vi "CSTK_BuildApplication_Manager_Package_Zip.vi"(5 "Files Generated by Build":path[](array[path]) caption="通过生成创建的文件", 7 "Destination Path":path caption="目标路径", 8 "error in (no error)":errorcluster caption="错误输入（无错误）", 10 "Build Specification Name":string caption="程序生成规范名称") -> (0 "error out":errorcluster caption="错误输出")   [LabVIEW 2015, in "CSTK_BuildApplication_Manager.lvlib"]
uses:
  CSTK_BuildApplication_Manager.lvlib
  CSTK_BuildApplication_Manager_data.ctl
  CSTK_BuildApplication_Manager_selector.ctl
  user32.dll
panel:
  in  "根据版本号修改EXE文件名":bool
  in  "打包成ZIP文件？":bool=TRUE
  in  "确定按钮":bool
  in  "注释":string
  # "Build Application Manager"
  # "输入版本修改日志"
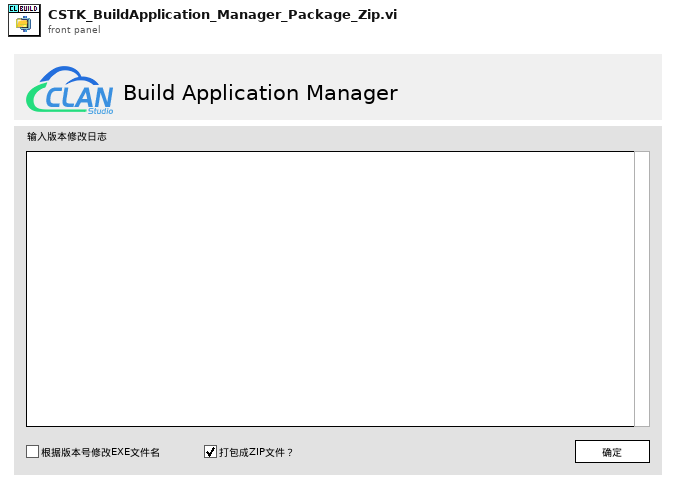
[diagram p1: front panel]
types:
  T1 = typedef "CSTK_BuildApplication_Manager.lvlib/CSTK_BuildApplication_Manager_data.ctl" = cluster{"Build Specification Name":string, "Destination Path":path, "Files Generated by Build":path[], "Exe Path Generated by Build":path, "Version":string, "Datatime":timestamp, "ChangeLog":string, "Package as a ZIP file?":bool, "Rename EXE File Name?":bool, "Zip File Path":path}
  T2 = enum32{"Invalid", "Standard", "Closed", "Hidden", "Minimized", "Maximized"}
  T3 = typedef "CSTK_BuildApplication_Manager.lvlib/CSTK_BuildApplication_Manager_selector.ctl" = cluster{"Package as a ZIP file?":bool, "Rename EXE File Name?":bool}
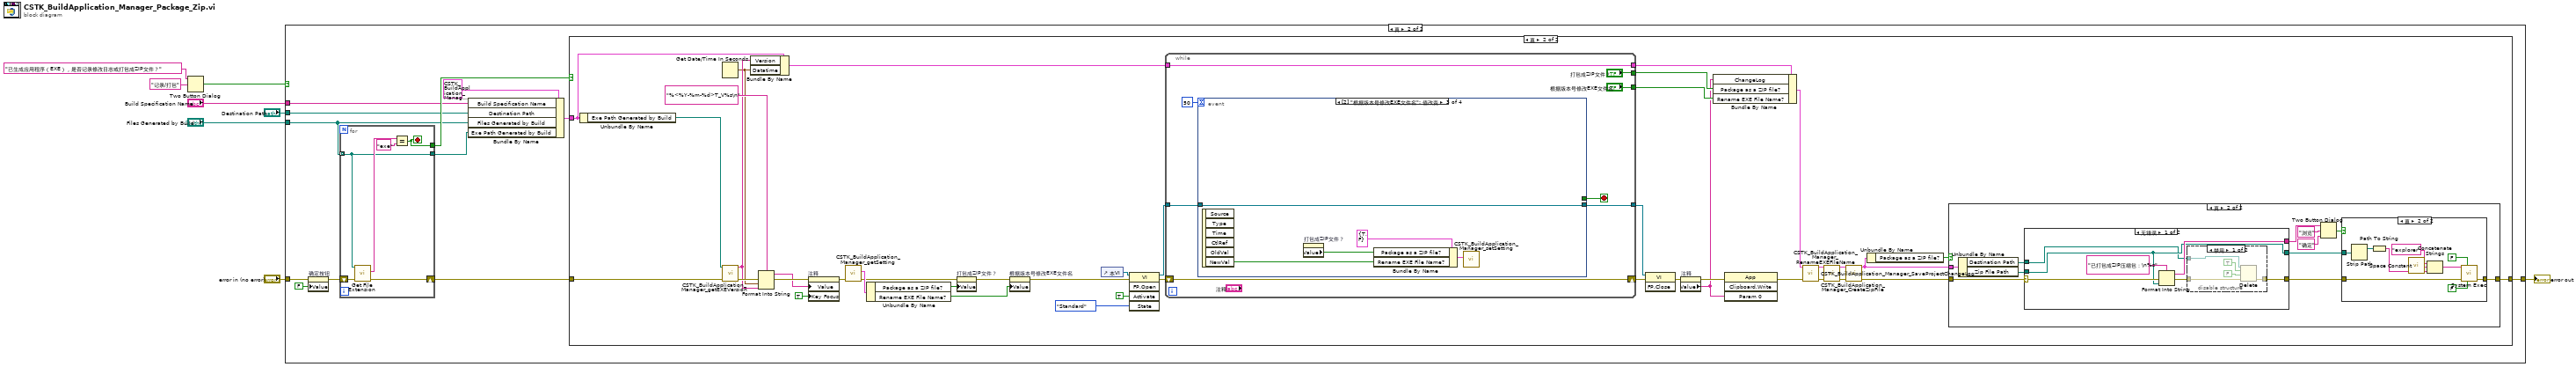
[diagram p0: block diagram]
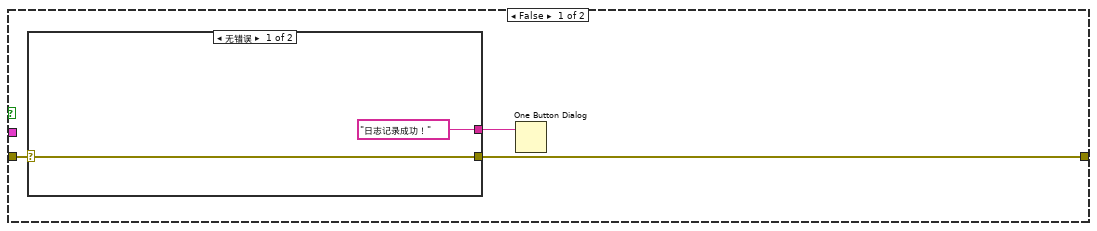
[diagram p4: hidden frame]
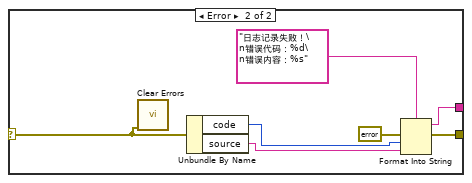
[diagram p5: hidden frame]
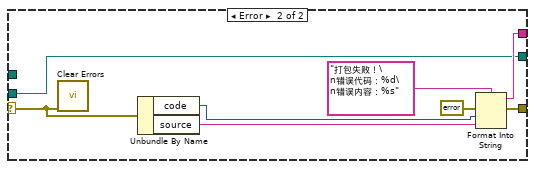
[diagram p8: hidden frame]
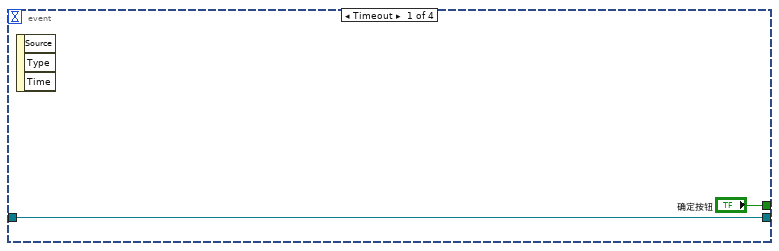
[diagram p9: hidden frame]
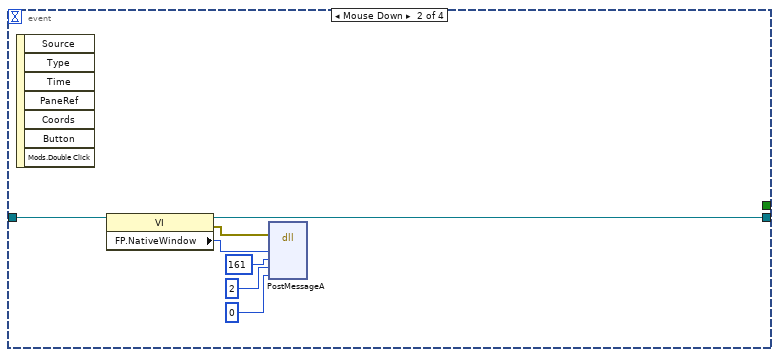
[diagram p10: hidden frame]
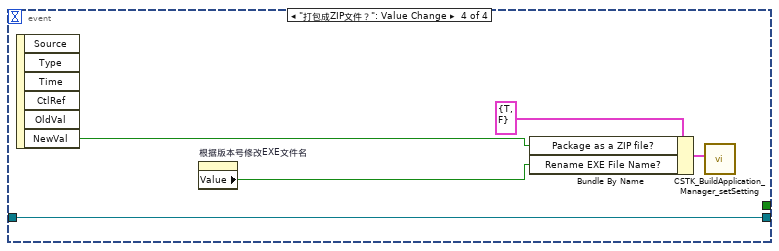
[diagram p11: hidden frame]
diagram:
  n1 = Two Button Dialog(message="已生成应用程序（EXE），是否记录修改日志或打包成ZIP文件？" ("消息"), 2:"记录/打包" ("T按钮名称（“确定”）")) -> (T button?=w1:bool)  [unwired: 1 in]
  n2 = case shown="真" w1 {
    tunnel: "Files Generated by Build" -> [_ w12]
    tunnel: "error in (no error)" -> [w9 w20]
    tunnel: [w9 w21] -> w5
    tunnel: "Build Specification Name" -> [_ w14]
    tunnel: "Destination Path" -> [_ w13]
    frame False {
    }
    frame True {
      n3 = property on="确定按钮" class="Bool (严格)"(error in=w20, "Value"=FALSE ("确定按钮")) -> (error out=w18:errorcluster)  [unwired: 1 in, 1 out]
      n4 = for {
        tunnel: w12 -> [w148] mode=indexing
        shift-right: [w146] -> w17
        shift-left: w18 -> [w151]
        tunnel: [w148] -> w11
        tunnel: [w147] -> w16
        stop <- w147 stop-if-true
        n5 = call <vilib>:"Get File Extension.vi"("error in (no error)"=w151, "file"=w148) -> ("error out"=w146:errorcluster, "lowercase file extension"=w150:string)  [unwired: 5 in, 3 out]
        n6 = Equal?(x=w150, y="exe") -> (x = y?=w147:bool)
      }
      n7 = Bundle By Name(cluster=T1 {"Build Specification Name"="", "Destination Path"=path "", "Files Generated by Build"=[], "Exe Path Generated by Build"=path "", "Version"="", "Datatime"=timestamp(0 s since 1904-01-01), "ChangeLog"="", "Package as a ZIP file?"=TRUE, "Rename EXE File Name?"=FALSE, "Zip File Path"=path ""} ("BuildApplication Data"), "Build Specification Name"=w14, "Destination Path"=w13, "Files Generated by Build"=w12, "Exe Path Generated by Build"=w11) -> (w10:T1)
      n8 = case shown="真" w16 {
        tunnel: [w22 w63] -> w21
        tunnel: w17 -> [w22 w62]
        tunnel: w10 -> [_ w44]
        frame False {
        }
        frame True {
          n9 = Unbundle By Name(w44) -> ("Exe Path Generated by Build"=w45:path)
          n10 = Get Date/Time In Seconds() -> (seconds since 1Jan1904=w42:timestamp)
          n11 = call "CSTK_BuildApplication_Manager_getEXEVersion.vi"("错误输入（无错误）"=w62, "EXE路径"=w45) -> ("错误输出"=w55:errorcluster, "版本号"=w43:string)  [unwired: 8 in]
          n12 = Bundle By Name(cluster=w44, "Version"=w43, "Datatime"=w42) -> (w41:T1)
          n13 = Format Into String(format string="%<%Y-%m-%d>T_V%s\n" ("格式字符串"), error in=w55, w42, w43) -> (resulting string=w53:string, error out=w54:errorcluster)  [unwired: 1 in]
          n14 = property on="注释" class="Str"(error in=w54, "Value"=w53, "Key Focus"=TRUE ("键选中")) -> (error out=w29:errorcluster)  [unwired: 1 in, 1 out]
          n15 = call "CSTK_BuildApplication_Manager_getSetting.vi"("Error in"=w29) -> ("Error out"=w23:errorcluster, "BuildApplication Selector"=w28:T3)  [unwired: 8 in, 1 out]
          n16 = Unbundle By Name(w28) -> ("Package as a ZIP file?"=w27:bool, "Rename EXE File Name?"=w26:bool)
          n17 = property on="打包成ZIP文件？" class="Bool (严格)"(error in=w23, "Value"=w27) -> (error out=w25:errorcluster)  [unwired: 1 in, 1 out]
          n18 = property on="根据版本号修改EXE文件名" class="Bool (严格)"(error in=w25, "Value"=w26) -> (error out=w24:errorcluster)  [unwired: 1 in, 1 out]
          n19 = control-ref of="本VI"() -> (w57:refnum<vi>)
          n20 = invoke class="VI" method="FP.Open"(reference=w57, error in=w24, "Activate"=TRUE ("激活？"), "State"=T2."Standard" ("状态")) -> (reference out=w47:refnum<vi>, error out=w59:errorcluster)  [unwired: 1 in, 3 out]
          n21 = while {
            shift-right: [w126] -> w58
            shift-left: w59 -> [w126]
            tunnel: ["打包成ZIP文件？"] -> w39
            tunnel: ["根据版本号修改EXE文件名"] -> w38
            tunnel: w47 -> [w120]
            tunnel: [w121] -> w46
            tunnel: w41 -> [w119]
            tunnel: [w119] -> w40
            stop <- w122 stop-if-true
            n22 = event shown="[2] \"根据版本号修改EXE文件名\": 值改变" {
              selector: _ -> [_ _ _ _]
              dyn-events: _ -> [_ _ _ _]
              timeout: 50 -> [_ _ _ _]
              tunnel: ["确定按钮" _ _ _] -> w122
              tunnel: [w127 w129 w140 w145] -> w121
              tunnel: w120 -> [w127 w130 w140 w145]
              event Timeout {
                n23 = event-data() -> ()  [unwired: 1 in, 3 out]
              }
              event Mouse Down {
                n24 = event-data() -> ()  [unwired: 1 in, 7 out]
                n25 = property class="VI"(reference=w130) -> (reference out=w129:refnum<vi>, error out=w131:errorcluster, "FP.NativeWindow"=w132:u64)  [unwired: 1 in]
                n26 = dll-call lib="user32.dll" fn="PostMessageA"(error in=w131, "hWnd"=w132, "Msg"=161, "wParam"=2, "IParam"=0 ("wParam")) -> ()  [unwired: 7 in, 2 out]
              }
              event "根据版本号修改EXE文件名": Value Change {
                n27 = event-data() -> ("NewVal"=w137:bool)  [unwired: 1 in, 5 out]
                n28 = property on="打包成ZIP文件？" class="Bool (严格)"() -> ("Value"=w136:bool)  [unwired: 2 in, 2 out]
                n29 = Bundle By Name(cluster=T3 {"Package as a ZIP file?"=TRUE, "Rename EXE File Name?"=FALSE} ("BuildApplication Selector"), "Package as a ZIP file?"=w136, "Rename EXE File Name?"=w137) -> (w138:T3)
                n30 = call "CSTK_BuildApplication_Manager_setSetting.vi"("BuildApplication Selector"=w138) -> ()  [unwired: 10 in, 1 out]
              }
              event "打包成ZIP文件？": Value Change {
                n31 = event-data() -> ("NewVal"=w141:bool)  [unwired: 1 in, 5 out]
                n32 = property on="根据版本号修改EXE文件名" class="Bool (严格)"() -> ("Value"=w142:bool)  [unwired: 2 in, 2 out]
                n33 = Bundle By Name(cluster=T3 {"Package as a ZIP file?"=TRUE, "Rename EXE File Name?"=FALSE} ("BuildApplication Selector"), "Package as a ZIP file?"=w141, "Rename EXE File Name?"=w142) -> (w143:T3)
                n34 = call "CSTK_BuildApplication_Manager_setSetting.vi"("BuildApplication Selector"=w143) -> ()  [unwired: 10 in, 1 out]
              }
            }
          }
          n35 = invoke class="VI" method="FP.Close"(reference=w46, error in=w58) -> (error out=w51:errorcluster)  [unwired: 1 in, 2 out]
          n36 = property on="注释" class="Str"(error in=w51) -> (error out=w50:errorcluster, "Value"=w36:string)  [unwired: 1 in, 1 out]
          n37 = Bundle By Name(cluster=w40, "ChangeLog"=w36, "Package as a ZIP file?"=w39, "Rename EXE File Name?"=w38) -> (w37:T1)
          n38 = invoke class="App" method="Clipboard.Write"(error in=w50, "Param 0"=w36) -> (error out=w48:errorcluster)  [unwired: 2 in, 3 out]
          n39 = call "CSTK_BuildApplication_Manager_RenameEXEFileName.vi"("错误输入（无错误）"=w48, "BuildApplication Data in"=w37) -> ("错误输出"=w49:errorcluster, "BuildApplication Data out"=w34:T1)  [unwired: 8 in]
          n40 = call "CSTK_BuildApplication_Manager_SaveProjectChangeLog.vi"("错误输入（无错误）"=w49, "BuildApplication Data in"=w34) -> ("错误输出"=w35:errorcluster, "BuildApplication Data out"=w33:T1)  [unwired: 8 in]
          n41 = call "CSTK_BuildApplication_Manager_CreateZipFile.vi"("错误输入（无错误）"=w35, "BuildApplication Data in"=w33) -> ("错误输出"=w32:errorcluster, "BuildApplication Data out"=w31:T1)  [unwired: 8 in]
          n42 = Unbundle By Name(w31) -> ("Package as a ZIP file?"=w30:bool)
          n43 = case shown="真" w30 {
            tunnel: [w65 w85] -> w63
            tunnel: w32 -> [w66 w83]
            tunnel: w31 -> [_ w78]
            frame False {
              n44 = case shown="无错误" w66 {
                selector: w66 -> [w68 w71]
                tunnel: [w68 w73] -> w65
                tunnel: ["日志记录成功！" ("格式字符串") w74] -> w64
                frame No Error {
                }
                frame Error {
                  n45 = call <vilib>:"Clear Errors.vi"("error in (no error)"=w71) -> ()  [unwired: 5 in, 2 out]
                  n46 = Unbundle By Name(w71) -> ("code"=w70:i32, "source"=w69:string)
                  n47 = Format Into String(format string="日志记录失败！\n错误代码：%d\n错误内容：%s" ("格式字符串"), error in=errorcluster {"status"=FALSE, "code"=0, "source"=""} ("错误输入"), w70, w69) -> (resulting string=w74:string, error out=w73:errorcluster)  [unwired: 1 in]
                }
              }
              n48 = One Button Dialog(message=w64) -> ()  [unwired: 1 in, 1 out]
            }
            frame True {
              n49 = Unbundle By Name(w78) -> ("Destination Path"=w76:path, "Zip File Path"=w77:path)
              n50 = case shown="无错误" w83 {
                selector: w83 -> [w103 w114]
                tunnel: w77 -> [w101 w111]
                tunnel: [w98 w116] -> w86
                tunnel: [w102 w117] -> w82
                tunnel: [w101 w111] -> w84
                tunnel: w76 -> [w100 _]
                frame No Error {
                  n51 = Format Into String(format string="已打包成ZIP压缩包：\n%s" ("格式字符串"), error in=w103, w101) -> (resulting string=w102:string, error out=w99:errorcluster)  [unwired: 1 in]
                  n52 = disable-structure shown="禁用" {
                    disable-tunnel: w100 -> [w109 _]
                    disable-tunnel: w99 -> [w106 w110]
                    disable-tunnel: [w105 w110] -> w98
                    frame Disabled {
                      n53 = Delete(path (use dialog)=w109, entire hierarchy (F)=TRUE ("整个层次结构(F)"), confirm (F)=FALSE ("确认(F)"), error in=w106) -> (error out=w105:errorcluster)  [unwired: 1 in, 2 out]
                    }
                    frame Enabled {
                    }
                  }
                }
                frame Error {
                  n54 = call <vilib>:"Clear Errors.vi"("error in (no error)"=w114) -> ()  [unwired: 5 in, 2 out]
                  n55 = Unbundle By Name(w114) -> ("code"=w113:i32, "source"=w112:string)
                  n56 = Format Into String(format string="打包失败！\n错误代码：%d\n错误内容：%s" ("格式字符串"), error in=errorcluster {"status"=FALSE, "code"=0, "source"=""} ("错误输入"), w113, w112) -> (resulting string=w117:string, error out=w116:errorcluster)  [unwired: 1 in]
                }
              }
              n57 = Two Button Dialog(message=w82, 1:"确定" ("F按钮名称（“取消”）"), 2:"浏览" ("T按钮名称（“确定”）")) -> (T button?=w81:bool)
              n58 = case shown="真" w81 {
                tunnel: [w87 w90] -> w85
                tunnel: w86 -> [w87 w91]
                tunnel: w84 -> [_ w94]
                frame False {
                }
                frame True {
                  n59 = Strip Path(path=w94) -> (stripped path=w93:path)  [unwired: 1 out]
                  n60 = Path To String(path=w93) -> (string=w95:string)
                  n61 = call <vilib>:"Space Constant.vi"() -> ("String"=w96:string)
                  n62 = Concatenate Strings("explorer" ("字符串"), w96, w95) -> (w92:string)
                  n63 = call <vilib>:"System Exec.vi"("run minimized? (F)"=FALSE, "wait until completion? (T)"=FALSE, "error in (no error)"=w91, "command line"=w92) -> ("error out"=w90:errorcluster)  [unwired: 4 in, 3 out]
                }
              }
            }
          }
        }
      }
    }
  }
  "error out" <- w5
